vi "Get Service Class Instances.vi"() -> (3 "service instances":refnum<class "ServiceBase.lvclass">[](array[class]))   [LabVIEW 2025, in "xnet_can_bus_monitor_api_server.lvlib"]
uses:
  xnet_can_bus_monitor_api_server.lvlib
  <vilib>/gRPC/LabVIEW gRPC Servicer/ServiceBase/ServiceBase.lvclass
  RPC Service/NI_XNET_CAN_Bus_Monitor_API/NI_XNET_CAN_Bus_Monitor_API.lvclass
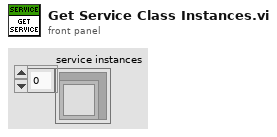
[diagram p1: front panel]
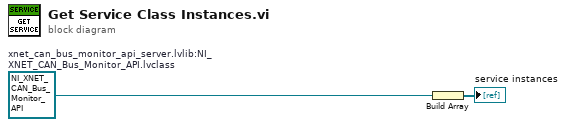
[diagram p0: block diagram]
diagram:
  w1 = refnum<class "NI_XNET_CAN_Bus_Monitor_API.lvclass"> refnum  # xnet_can_bus_monitor_api_server.lvlib:NI_XNET_CAN_Bus_Monitor_API.lvclass
  n1 = Build Array(w1) -> (→"service instances":refnum<class "NI_XNET_CAN_Bus_Monitor_API.lvclass">[])
